vi "To String.vi"(8 "error in (no error)":errorcluster, 10 "Parameters":variant, 11 "DataSingleElement in":refnum<class "DataSingleElement.lvclass">) -> (0 "error out":errorcluster, 2 "String":string, 3 "DataSingleElement out":refnum<class "DataSingleElement.lvclass">)   [LabVIEW 2014, in "DataSingleElement.lvclass"]
uses:
  DataSingleElement.lvclass
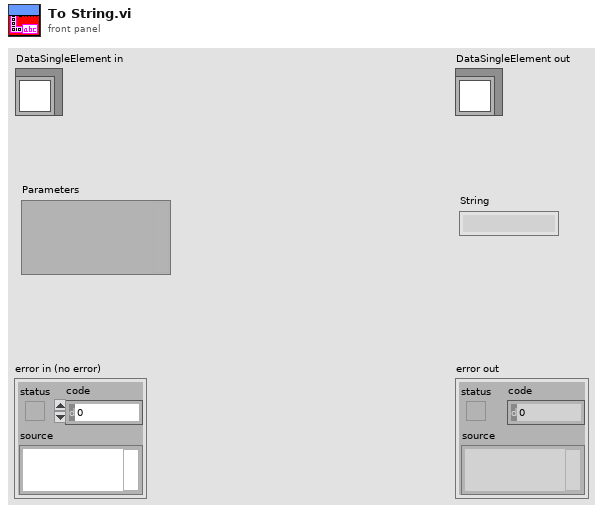
[diagram p1: front panel]
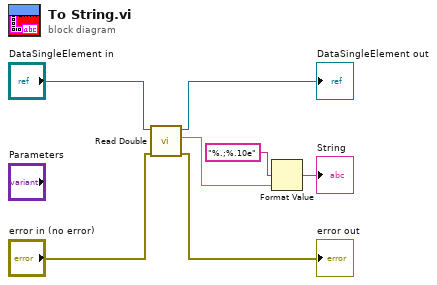
[diagram p0: block diagram]
diagram:
  n1 = call "Read Double.vi"("error in (no error)"="error in (no error)", "DataSingleElement in"="DataSingleElement in") -> ("error out"=→"error out":errorcluster, "value"=w5:dbl, "DataSingleElement out"=→"DataSingleElement out":refnum<class "DataSingleElement.lvclass">)  [unwired: 7 in]
  n2 = Format Value(format string="%.;%.10e", value (0)=w5) -> (output string=→"String":string)  [unwired: 1 in]
